vi "Log Strain.vi"(8 "error in (no error)":errorcluster, 10 "Input file":path=path "\\\\myhome\\NHMFL/RAW_DATA/Collected Strain Data/p_c3_012_091724.tdms", 11 "Strain Logger in":refnum<class "Strain Logger.lvclass">) -> (0 "error out":errorcluster, 3 "Strain Logger out":refnum<class "Strain Logger.lvclass">)   [LabVIEW 2024, in "Strain Logger.lvclass"]
uses:
  Strain Logger.lvclass
  <vilib>/Utility/error.llb/Error Cluster From Error Code.vi
  <vilib>/ErrorRing/Error Ring.xnode
panel:
  in  "Field chan":string="Field"
  out "found":bool
  out "Parameters":dbl[][](array[numeric])
  out "Array":string[](array[string])
  out "File time stamp":timestamp
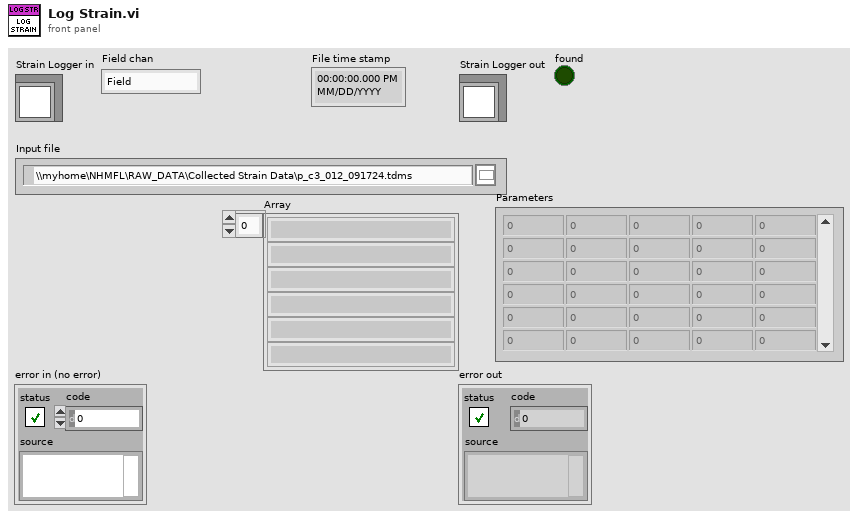
[diagram p1: front panel]
types:
  T1 = enum16{"open", "open or create", "create or replace", "create", "open (read-only)"}
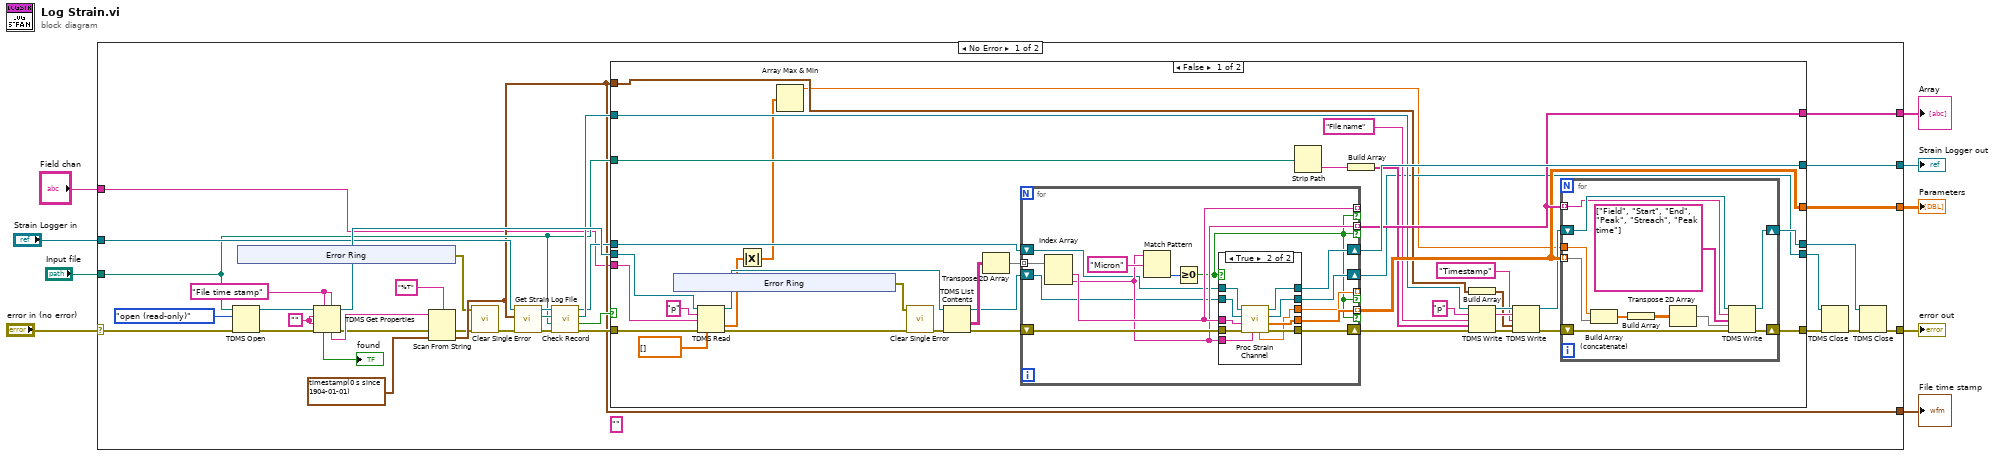
[diagram p0: block diagram]
diagram:
  n1 = case shown="No Error" "error in (no error)" {
    selector: "error in (no error)" -> [w40 w133]
    tunnel: [w27 w133] -> w8
    tunnel: [w37 w132] -> w6
    tunnel: "Strain Logger in" -> [w36 w132]
    tunnel: "Input file" -> [w24 _]
    tunnel: [w15 _] -> w4
    tunnel: [w38 _] -> w3
    tunnel: [w31 _] -> w2
    tunnel: "Field chan" -> [w10 _]
    frame No Error {
      (unwired) "" ("format string")
      w20 = ""
      w19 = "File time stamp" ("property name")
      n2 = TDMS Open(8:w40, 10:T1."open (read-only)" ("operation (0:open)"), 11:w24) -> (0:w42:errorcluster, 3:w43:refnum<k34>)  [unwired: 4 in]
      n3 = xnode "Error Ring"() -> ("error out"=w11:errorcluster)
      n4 = TDMS Get Properties(5:w19, 7:w19, 8:w42, 9:w20, 10:w20, 11:w43) -> (0:w16:errorcluster, 3:w39:refnum<k34>, 4:w18:string, 6:→"found":bool)  [unwired: 2 out]
      n5 = Scan From String(format string="%T", input string=w18, error in=w16, default 1=timestamp(0 s since 1904-01-01)) -> (error out=w13:errorcluster, output 1=w15:timestamp)  [unwired: 1 in, 2 out]
      n6 = call "Clear Single Error.vi"("Error In"=w13, "Error to clear"=w11) -> ("Error Out"=w12:errorcluster)  [unwired: 8 in, 1 out]
      n7 = call-dynamic "Get Strain Log File.vi"("error in (no error)"=w12, "Time Stamp"=w15, "Strain Logger in"=w36) -> ("error out"=w33:errorcluster, "Log file name"=w34:path, "Strain Logger out"=w35:refnum<class "Strain Logger.lvclass">)  [unwired: 6 in]
      n8 = call-dynamic "Check Record.vi"("error in (no error)"=w33, "Pulse file name"=w24, "Log file name"=w34, "Strain Logger in"=w35) -> ("error out"=w32:errorcluster, "Record exists"=w30:bool, "tdms file out"=w25:refnum<k34>, "Strain Logger out"=w23:refnum<class "Strain Logger.lvclass">)  [unwired: 4 in]
      n9 = case shown="False" w30 {
        tunnel: w39 -> [w58 w130]
        tunnel: [w79 _] -> w38
        tunnel: [w81 w128] -> w37
        tunnel: w23 -> [w80 w128]
        tunnel: w32 -> [w59 w131]
        tunnel: [w78 _] -> w31
        tunnel: [w63 w131] -> w22
        tunnel: [w62 w130] -> w29
        tunnel: [w64 w129] -> w26
        tunnel: w25 -> [w76 w129]
        tunnel: w24 -> [w61 _]
        tunnel: w15 -> [w68 _]
        tunnel: w10 -> [w55 _]
        frame False {
          n10 = xnode "Error Ring"() -> ("error out"=w48:errorcluster)
          n11 = TDMS Read(0:w58, 5:"p" ("group name in"), 7:w55, 11:w59, 12:dbl[] []) -> (4:w57:refnum<k34>, 10:w53:dbl[], 15:w50:errorcluster)  [unwired: 3 in, 3 out]
          n12 = Absolute Value(x=w53) -> (abs(x)=w52:dbl[])
          n13 = Array Max & Min(array=w52) -> (max value=w51:dbl)  [unwired: 3 out]
          n14 = call "Clear Single Error.vi"("Error In"=w50, "Error to clear"=w48) -> ("Error Out"=w49:errorcluster)  [unwired: 8 in, 1 out]
          n15 = TDMS List Contents(4:w49, 7:w57) -> (0:w83:errorcluster, 1:w85:string[][], 3:w82:refnum<k34>)  [unwired: 1 in, 1 out]
          n16 = Transpose 2D Array(2D array=w85) -> (transposed array=w84:string[][])
          n17 = for {
            tunnel: w84 -> [w112] mode=indexing
            tunnel: [w108] -> w79 mode=indexing if=w101
            tunnel: [w109] -> _ mode=indexing if=w101
            shift-right: [w110] -> w77
            shift-left: w83 -> [w111]
            shift-right: [w106] -> w62
            shift-left: w82 -> [w107]
            shift-right: [w104] -> w81
            shift-left: w80 -> [w105]
            tunnel: [w103] -> w78 mode=indexing if=w101
            tunnel: [w102] -> _ mode=indexing if=w101
            n18 = Index Array(array=w112) -> (element #1=w109:string, element #2=w108:string)  [unwired: 2 in]
            n19 = Match Pattern(string=w108, regular expression="Micron" ("search string")) -> (offset past match=w113:i32)  [unwired: 1 in, 3 out]
            n20 = Greater Or Equal To 0?(x=w113) -> (x >= 0?=w101:bool)
            n21 = case shown="True" w101 {
              tunnel: w111 -> [w117 w127]
              tunnel: [w117 w126] -> w110
              tunnel: w109 -> [_ w125]
              tunnel: w108 -> [_ w124]
              tunnel: w107 -> [w116 w123]
              tunnel: [w116 w122] -> w106
              tunnel: w105 -> [w115 w121]
              tunnel: [w115 w120] -> w104
              tunnel: [_ w119] -> w103
              tunnel: [_ w118] -> w102
              frame False {
              }
              frame True {
                n22 = call-dynamic "Proc Strain Channel.vi"("channel name"=w124, "error in (no error)"=w127, "group name in"=w125, "tdms file"=w123, "Strain Logger in"=w121) -> ("error out"=w126:errorcluster, "Parameters"=w119:dbl[], "tdms file out"=w122:refnum<k34>, "Strain Logger out"=w120:refnum<class "Strain Logger.lvclass">, "Max time"=w118:dbl)  [unwired: 2 in]
              }
            }
          }
          n23 = Strip Path(path=w61) -> (name=w60:string)  [unwired: 1 out]
          n24 = Build Array(w60) -> (w73:string[])
          n25 = Build Array(w68) -> (w67:timestamp[])
          n26 = TDMS Write(0:w76, 5:"p" ("group name in (Untitled)"), 7:"File name" ("group name in (Untitled)"), 9:w73, 11:w77) -> (4:w71:refnum<k34>, 6:w70:string, 15:w72:errorcluster)  [unwired: 1 in, 1 out]
          n27 = TDMS Write(0:w71, 5:w70, 7:"Timestamp" ("group name in (Untitled)"), 9:w67, 11:w72) -> (4:w65:refnum<k34>, 15:w66:errorcluster)  [unwired: 1 in, 2 out]
          n28 = for {
            tunnel: w79 -> [w95] mode=indexing
            tunnel: w78 -> [w100] mode=indexing
            shift-right: [w96] -> w63
            shift-left: w66 -> [w99]
            shift-right: [w97] -> w64
            shift-left: w65 -> [w98]
            tunnel: w51 -> [w92]
            n29 = Build Array (concatenate)(w92, w100) -> (w91:dbl[])
            n30 = Build Array(w91) -> (w90:dbl[][])
            n31 = Transpose 2D Array(2D array=w90) -> (transposed array=w93:dbl[][])
            n32 = TDMS Write(0:w98, 5:w95, 7:string[] ["Field", "Start", "End", "Peak", "Streach", "Peak time"] ("channel name(s) in (Untitled)"), 9:w93, 11:w99) -> (4:w97:refnum<k34>, 15:w96:errorcluster)  [unwired: 1 in, 2 out]
          }
        }
        frame True {
        }
      }
      n33 = TDMS Close(8:w22, 11:w29) -> (0:w28:errorcluster)  [unwired: 1 out]
      n34 = TDMS Close(8:w28, 11:w26) -> (0:w27:errorcluster)  [unwired: 1 out]
    }
    frame Error {
    }
  }
  "error out" <- w8
  "Strain Logger out" <- w6
  "File time stamp" <- w4
  "Array" <- w3
  "Parameters" <- w2
